vi "calibrationElectrometer_monitorCommand_stopScan.vi"(8 "error in (no error)":errorcluster, 11 "command_stopScan_Ctl":T1) -> (0 "error out":errorcluster, 2 "function return":i32, 3 "command_stopScan_Ctl out":T1)   [LabVIEW 2016, in "SALLV_calibrationElectrometer.lvlib"]
doc: "int calibrationElectrometer_shm_monitorCommand_stopScanLV(calibrationElectrometer_command_stopScanLV *command_stopScan_Ctl );"
uses:
  SALLV_calibrationElectrometer.lvlib
  DataTypes/command_stopScan.ctl
  SALLV_calibrationElectrometer.so
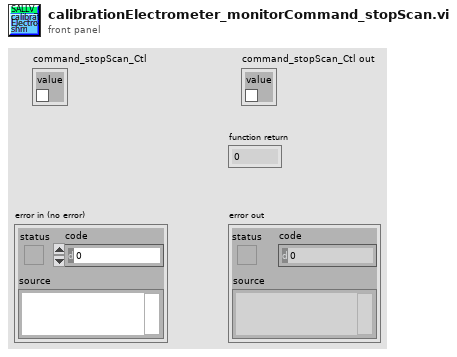
[diagram p1: front panel]
types:
  T1 = typedef "SALLV_calibrationElectrometer.lvlib/command_stopScan.ctl" = cluster{"value":bool}
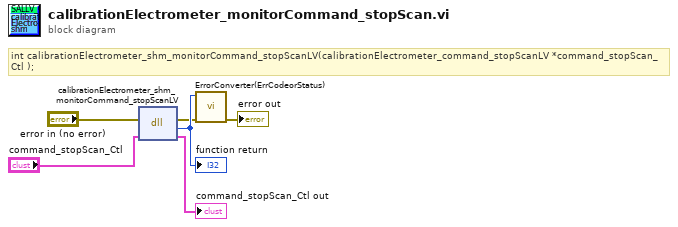
[diagram p0: block diagram]
diagram:
  # "int calibrationElectrometer_shm_monitorCommand_stopScanLV(calibrationElectrometer_command_stopScanLV *command_stopScan_Ctl );"
  n1 = dll-call lib="home/andres/Desktop/SAL_calibrationElectrometer/SALLV_calibrationElectrometer.*" fn="calibrationElectrometer_shm_monitorCommand_stopScanLV"(error in="error in (no error)", "command_stopScan_Ctl"="command_stopScan_Ctl") -> (error out=w2:errorcluster, w6:i32, "command_stopScan_Ctl"=→"command_stopScan_Ctl out":T1)  [unwired: 2 in, 1 out]
  "function return" <- w6
  n2 = call "ErrorConverter(ErrCodeorStatus).vi"("error in (no error)"=w2, "error code"=w6) -> ("error out"=→"error out":errorcluster)  [unwired: 9 in]
